vi "Global_ShooterCTRL.vi"() -> ()   [LabVIEW 2017]
panel:
  in  "Hopper Feed CTRL":dbl
  in  "Hood Pos/Vbus":bool
  in  "Hood VBUS CTRL":dbl
  in  "Fly Wheel CTRL":dbl
  in  "Hood Position CTRL":dbl
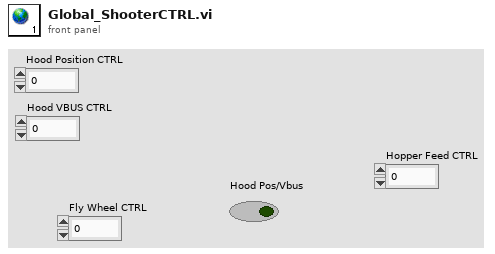
[diagram p1: front panel]
diagram:
